vi "Kinect Create.vi"(11 "Depth Format":i32(ring)=1 items=["Undefined", "Resolution640x480Fps30", "Resolution320x240Fps30", "Resolution80x60Fps30"]) -> (0 "error out":errorcluster)   [LabVIEW 2011]
uses:
  <vilib>/vision/Image Controls.llb/IMAQ Image.ctl
  Microsoft.Kinect
  Kinect Global Status.vi
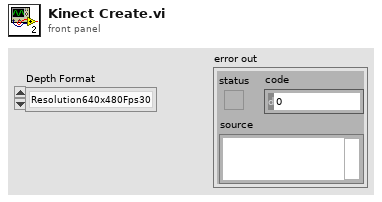
[diagram p1: front panel]
types:
  T1 = typedef "IMAQ Image.ctl" = refnum<image>
  T2 = cluster{"Image Height":i32, "Image Width":i32, "Minimum Framerate":i32, "Maximum Framerate":i32, "Framerate":i32, "Near Mode":bool, "Range":sgl}
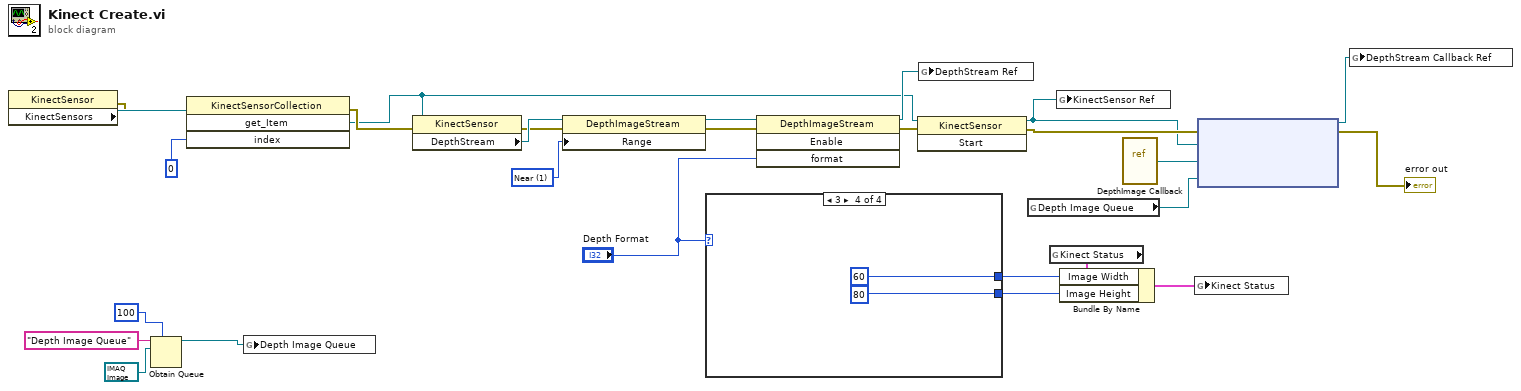
[diagram p0: block diagram]
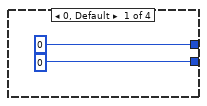
[diagram p2: hidden frame]
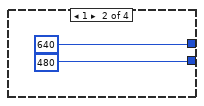
[diagram p3: hidden frame]
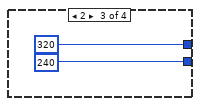
[diagram p4: hidden frame]
diagram:
  w8 = 1 items=["Default", "Near"] ("Range")
  n1 = property class="KinectSensor"() -> (error out=w25:errorcluster, "KinectSensors"=w27:refnum<k24>)  [unwired: 2 in, 1 out]
  n2 = Obtain Queue(max queue size (-1, unlimited)=100, name (unnamed)="Depth Image Queue", element data type=T1 refnum ("New Image")) -> (queue out=w12:refnum<queue>)  [unwired: 2 in, 2 out]
  n3 = invoke class="KinectSensorCollection" method="get_Item"(reference=w27, error in=w25, "index"=0) -> (error out=w24:errorcluster, "get_Item"=w11:refnum<k24>)  [unwired: 1 in, 2 out]
  n4 = global write "Kinect Global Status.vi" "Depth Image Queue"(w12) -> ()
  n5 = property class="KinectSensor"(reference=w11, error in=w24) -> (error out=w9:errorcluster, "DepthStream"=w10:refnum<k24>)  [unwired: 1 out]
  n6 = property class="DepthImageStream"(reference=w10, error in=w9, "Range"=w8) -> (reference out=w7:refnum<k24>, error out=w6:errorcluster)
  n7 = case shown="3" "Depth Format" {
    tunnel: [0 640 320 60] -> w2
    tunnel: [0 480 240 80] -> w1
    frame 0, Default {
    }
    frame 1 {
    }
    frame 2 {
    }
    frame 3 {
    }
  }
  n8 = invoke class="DepthImageStream" method="Enable"(reference=w7, error in=w6, "format"="Depth Format") -> (reference out=w18:refnum<k24>, error out=w23:errorcluster)  [unwired: 1 in, 2 out]
  n9 = invoke class="KinectSensor" method="Start"(reference=w11, error in=w23) -> (reference out=w17:refnum<k24>, error out=w21:errorcluster)  [unwired: 1 in, 1 out]
  n10 = global write "Kinect Global Status.vi" "DepthStream Ref"(w18) -> ()
  n11 = global read "Kinect Global Status.vi" "Depth Image Queue"() -> (w22:refnum<queue>)
  n12 = global read "Kinect Global Status.vi" "Kinect Status"() -> (w5:T2)
  n13 = global write "Kinect Global Status.vi" "KinectSensor Ref"(w17) -> ()
  n14 = Bundle By Name(cluster=w5, "Image Width"=w2, "Image Height"=w1) -> (w4:T2)
  n15 = vi-ref "DepthImage Callback.vi"() -> ("vi reference"=w20:refnum<vi>)
  n16 = global write "Kinect Global Status.vi" "Kinect Status"(w4) -> ()
  n17 = node(w21, w17, w20, w22) -> (w16:refnum<k27>, →"error out":errorcluster)  [unwired: 1 in]
  n18 = global write "Kinect Global Status.vi" "DepthStream Callback Ref"(w16) -> ()
